vi "Test_Adam_Out_Loop.vi"(9 "Array":bool[](array[boolean])=[FALSE, FALSE, FALSE, FALSE, FALSE, FALSE, FALSE, FALSE], 10 "Address (1)":u8=1, 11 "VISA name":refnum<visa-resource-name>="COM1") -> ()   [LabVIEW 2016]
panel:
  out "Adam_Out_Error":bool=TRUE
  out "F1_CO_On":bool
  out "F2_CO_On":bool
  out "TGA_Gas_select":bool
  in  "Adam_Out_FB":u16
  in  "stop":bool
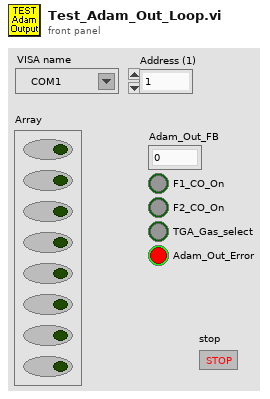
[diagram p1: front panel]
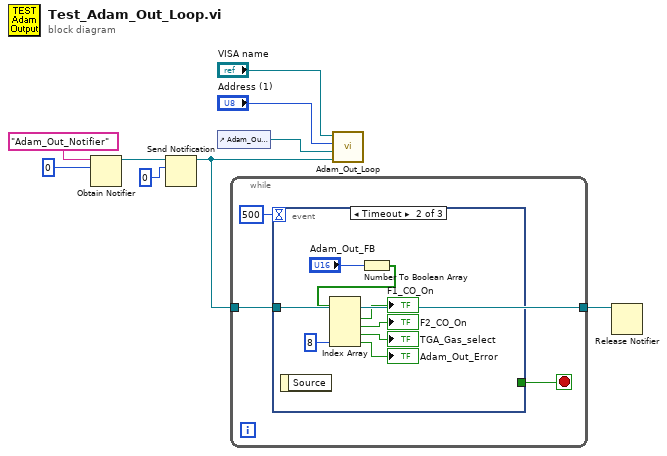
[diagram p0: block diagram]
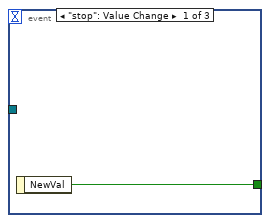
[diagram p2: hidden frame]
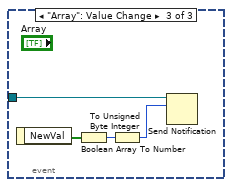
[diagram p3: hidden frame]
diagram:
  n1 = Obtain Notifier(name (unnamed)="Adam_Out_Notifier", notification data type=u8 0) -> (notifier out=w4:refnum<notifier>)  [unwired: 2 in, 2 out]
  n2 = Send Notification(notification=u8 0, notifier=w4) -> (notifier out=w3:refnum<notifier>)  [unwired: 1 in, 1 out]
  n3 = control-ref of="Adam_Out_FB"() -> (w1:refnum<vi>)
  n4 = while {
    tunnel: w3 -> [w11]
    tunnel: [w11] -> w5
    stop <- w12 stop-if-true
    n5 = event shown="[1] Timeout" {
      selector: _ -> [_ _ _]
      dyn-events: _ -> [_ _ _]
      timeout: 500 -> [_ _ _]
      tunnel: [w13 _ _] -> w12
      tunnel: w11 -> [_ _ w23]
      event "stop": Value Change {
        n6 = event-data() -> ("NewVal"=w13:bool)  [unwired: 1 in]
      }
      event Timeout {
        n7 = event-data() -> ()  [unwired: 1 in, 1 out]
        n8 = Number To Boolean Array(number="Adam_Out_FB") -> (Boolean array=w14:bool[])
        n9 = Index Array(array=w14, index #4=8 ("index")) -> (element #1=→"F1_CO_On":bool, element #2=→"F2_CO_On":bool, element #3=→"TGA_Gas_select":bool, element #4=→"Adam_Out_Error":bool)  [unwired: 3 in]
      }
      event "Array": Value Change {
        n10 = event-data() -> ("NewVal"=w24:bool[])  [unwired: 1 in]
        n11 = Boolean Array To Number(Boolean array=w24) -> (number=w22:u32)
        n12 = To Unsigned Byte Integer(number=w22) -> (unsigned 8bit integer=w21:u8)
        n13 = Send Notification(notification=w21, notifier=w23) -> ()  [unwired: 1 in, 2 out]
      }
    }
  }
  n14 = call "Adam_Out_Loop.vi"("Adam_Out_Notifier"=w3, "OP_feedback_ref"=w1, "Address (1)"="Address (1)", "VISA name"="VISA name") -> ()  [unwired: 7 in, 1 out]
  n15 = Release Notifier(notifier=w5) -> ()  [unwired: 2 in, 3 out]
